vi "Main.vi"() -> ()   [LabVIEW 2018]
uses:
  Shared Dependencies/Grouping Control.ctl
  Shared Dependencies/Container - Regex array.ctl
  Shared Dependencies/Shared Dependencies.lvlib
  Name and Dependency processing/Name and Dependency Processing.lvlib
panel:
  in  "Container - Regex pairs":T1=[{"Container to create"="TEST", "Regex"="^test_.*\\.vi"}, {"Container to create"="TEST", "Regex"="_test.vi$"}, {"Container to create"="DRV", "Regex"="^DRV_.*\\.lv.*$"}, {"Container to create"="HWT", "Regex"="^HWT_.*\\.lv.*$"}, {"Container to create"="FCN", "Regex"="^FCN_.*\\.lv.*$"}, {"Container to create"="INS", "Regex"="^INS_.*\\.lv.*$"}]
  in  "Groupings":T2={"Group vi.lib"=FALSE, "Group instr.lib"=FALSE, "Group user.lib"=FALSE, "Group All LabVIEW"=FALSE, "Make Custom Containers"=TRUE, "Ignore LabVIEW directory"=TRUE}
  in  "Create Unowned Container?":bool=TRUE
  in  "Input Folder Path":path=path "P:/sandbox/Ins_ExampleInstr_18.4_trunk"
  in  "Output File":path
  # "Arrows point TO dependency!  (i.e. Caller points TO Callee)"
  # "Grouping by vi.lib, instr.lib, user.lib and All LabVIEW is currently not implented. Custom containers and \"Ignore LabVIEW\" are."
  # "This is for creating custom containers based on filenames (not paths). \nFor example, the first two will group \"test_... and ..._test\" in to the same container."
  # "<---"
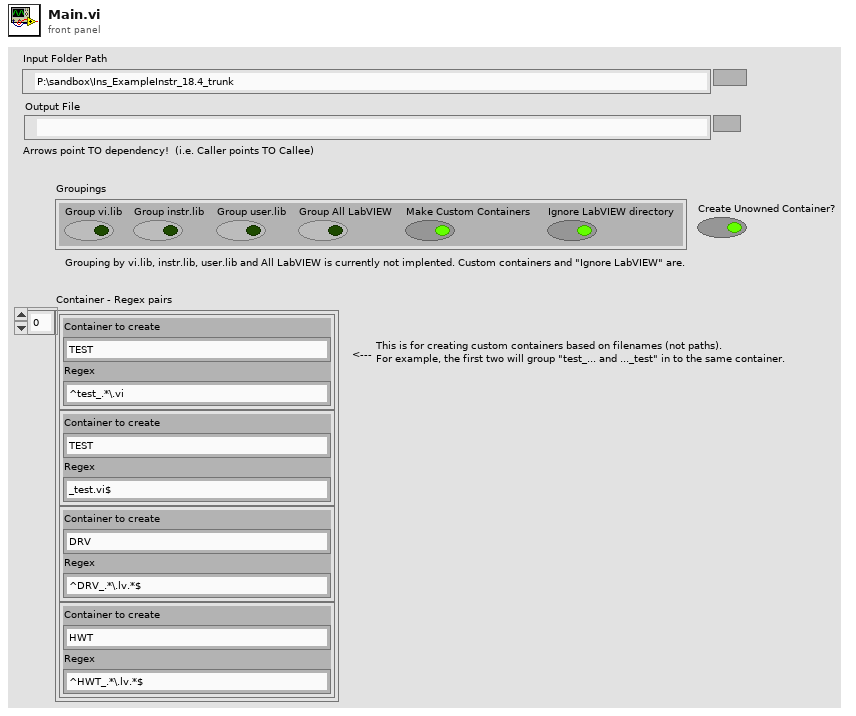
[diagram p1: front panel]
types:
  T1 = typedef "Shared Dependencies.lvlib/Container - Regex array.ctl" = cluster{"Container to create":string, "Regex":string}[]
  T2 = typedef "Name and Dependency Processing.lvlib/Grouping Control.ctl" = cluster{"Group vi.lib":bool, "Group instr.lib":bool, "Group user.lib":bool, "Group All LabVIEW":bool, "Make Custom Containers":bool, "Ignore LabVIEW directory":bool}
  T3 = typedef "Name and Dependency Processing.lvlib/Name - Dep Cluster.ctl" = cluster{"Name":string, "Dependency Names":string[]}
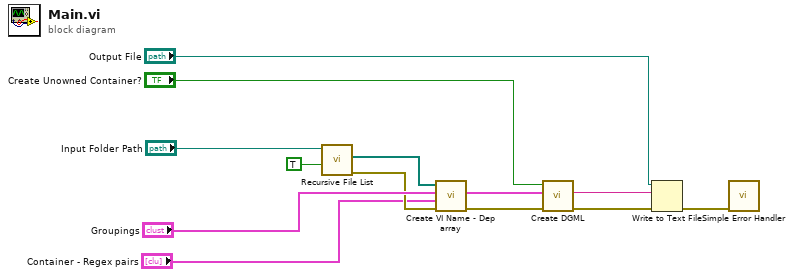
[diagram p0: block diagram]
diagram:
  n1 = call <vilib>:"Recursive File List.vi"("Continue Recursing on Error? (F)"=TRUE ("Treat LLBs as Folders?"), "Folder Path"="Input Folder Path") -> ("error out"=w4:errorcluster, "All Files in Dir"=w7:path[])  [unwired: 5 in, 3 out]
  n2 = call "Create VI Name - Dep array.vi"("error in (no error)"=w4, "Container - Regex pairs"="Container - Regex pairs", "Groupings"="Groupings", "All Files in Dir"=w7) -> ("error out"=w2:errorcluster, "Name-Dep Array"=w10:T3[])  [unwired: 6 in]
  n3 = call "Create DGML.vi"("error in (no error)"=w2, "Array"=w10, "Create Unowned Container?"="Create Unowned Container?") -> ("error out"=w8:errorcluster, "DGML File"=w6:string)  [unwired: 7 in]
  n4 = Write to Text File(file (use dialog)="Output File", text=w6, error in=w8) -> (error out=w5:errorcluster)  [unwired: 1 in, 2 out]
  n5 = call <vilib>:"Simple Error Handler.vi"("error in (no error)"=w5) -> ()  [unwired: 4 in, 5 out]
